vi "Control Type.vi"(11 "Valve in":refnum<class "MultiControl.lvclass">) -> (2 "Valve Type":string)   [LabVIEW 2020, in "VolatusControl.lvlib" / "MultiControl.lvclass"]
uses:
  MultiControl.lvclass
  MultiControl.lvclass/MultiControl.ctl
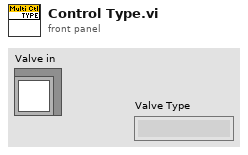
[diagram p1: front panel]
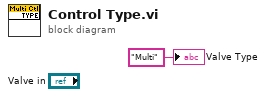
[diagram p0: block diagram]
diagram:
  "Valve Type" <- "Multi" ("Valve Type")
